vi "ElevatorSim_Execute.vi"(5 "LinearSystemID_Elevator_Model _Params":T7={"DCMOTOR_TYPES"=enum."NEO", "Num Motors"=1, "WinchRadias_Meters"=0.75, "mass_Kg"=26.0, "Gearing"=128.0} {"Gearing" format="%#_13g"; "mass_Kg" format="%#_13g"; "WinchRadias_Meters" format="%#_13g"}, 7 "ElevatorSim_Simulation _Params":T6={"MinHeight_Meters"=0.0, "MaxHeight_Meters"=0.0, "Measurment StdDev"=0.09, "SimulateGravity"=TRUE} {"Measurment StdDev" format="%#_13g"}, 8 "dT_Seconds":dbl=0.02 format="%#_13g", 10 "Battery Volts":dbl=12.0, 11 "Motor Dmd":dbl) -> (0 "Error":bool, 1 "AtLowLimit":bool, 2 "At HIgh LImit":bool, 3 "ElevatorHeight_Meters":dbl, 4 "Motor Current":dbl, 6 "out ElevatorSim":T1={"LinearSystemSim"={"m_Plant"={"m_A"=[], "m_B"=[], "m_C"=[], "m_D"=[], "States"=0, "Inputs"=0, "Outputs"=0}, "m_X"=[], "m_Y"=[], "m_U"=[], "MeasureStdDev"=[]}, "GearBox"={"nominalVoltage_Volts"=0.0, "StallTorque_NM"=0.0, "StallCurrent_Amps"=0.0, "FreeCurrent_Amps"=0.0, "FreeSpeed_RadPerSec"=0.0, "R_Ohms"=0.0, "KvINV_RadPerSecPerVolt"=0.0, "Kt_NMPerAmp"=0.0, "L_H"=0.0, "Jr_KgM2"=0.0}, "Gearing"=0.0, "DrumRadius_M"=0.0, "MinHeight_M"=0.0, "MaxHeight_M"=0.0, "CarriageMass_Kg"=0.0, "SimulateGravity"=TRUE} {"GearBox"."Jr_KgM2" format="%13.5p"; "GearBox"."L_H" format="%13.5p"; "GearBox"."Kt_NMPerAmp" format="%13.5p"; "GearBox"."KvINV_RadPerSecPerVolt" format="%13.5p"; "GearBox"."R_Ohms" format="%13.5p"; "GearBox"."FreeSpeed_RadPerSec" format="%13.5p"; "GearBox"."FreeCurrent_Amps" format="%13.5p"; "GearBox"."StallCurrent_Amps" format="%13.5p"; "GearBox"."StallTorque_NM" format="%13.5p"; "GearBox"."nominalVoltage_Volts" format="%13.5p"})   [LabVIEW 2019, in "Trajectory_Library.lvlib"]
doc: "Single call LabVIEW function to simulate an Elevatorr system. \n\nThe Elevator linear system definition is:\n - States\n - position (meters)\n - velocity (meters/sec)\n - Inputs:\n - motor voltage (volts)\n - Outputs:\n - position (meters)\n\n\nInputs:\n - LinearSystem Elevator Model Params -- cluster -- Contains physical configuration for Elevator system.\n - Elevator Sim Simulation Params -- cluster -- Contains siulation configuration.\n - Motor Dmd (CO) -- double -- motor demand value (+/- 1.0 )\n - Battery Voltage -- double -- Current simulated battery voltage (Volts)\n - dT Sec -- double -- Update period (Seconds, Default: 0.02)\n\nOutputs:\n - ElevatorHeight -- double -- Current elevator height (meters)\n - At High Limit -- boolean -- Elevator has reached high height limit\n - At Low Limit -- boolean -- Elevator has reached low height limit\n - Error -- boolean -- If TRUE an error occured.\n - Motor Current -- double -- Current motor current (Amps)\n - outElevatorSim -- cluster -- Current internal data cluster."
uses:
  Trajectory_Library.lvlib
  <vilib>/Analysis/Matrix/Datatypes/RealMatrix.ctl
  <vilib>/Analysis/Matrix/NI_Matrix.lvlib
  TypeDef/LINEAR_SYSTEM.ctl
  Enum/DCMOTOR_TYPES_ENUM.ctl
  TypeDef/LINEAR_SYSTEM_SIM.ctl
  TypeDef/DCMOTOR.CTL
  TypeDef/ELEVATOR_SIM.ctl
  TypeDef/LINEAR_SYSTEM_ID_ELEVATOR_MODEL.CTL
  TypeDef/ELEVATOR_SIM_SIMULATION_PARAMS.ctl
panel:
  out "Velocity_MetersPerSec":dbl
  # "<States, 1>"
  # "<Outputs, 1>"
  # "<Inputs, 1>"
  # "<Outputs, 1>"
  # "<States,States>"
  # "<States,Inputs>"
  # "<Outputs,States>"
  # "<Outputs,Inputs>"
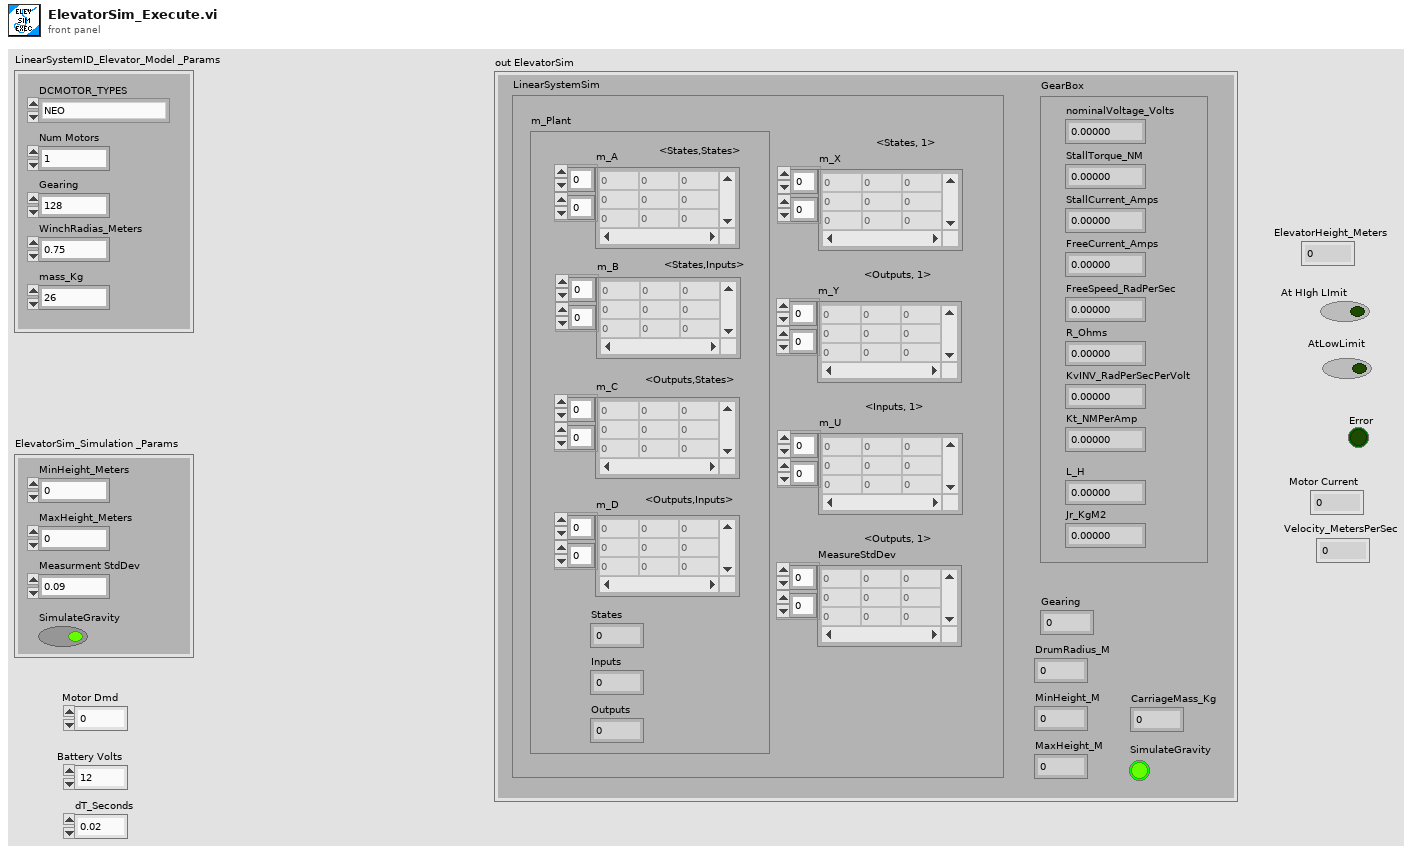
[diagram p1: front panel]
types:
  T1 = typedef "Trajectory_Library.lvlib/ELEVATOR_SIM.ctl" = cluster{"LinearSystemSim":T2, "GearBox":T5, "Gearing":dbl, "DrumRadius_M":dbl, "MinHeight_M":dbl, "MaxHeight_M":dbl, "CarriageMass_Kg":dbl, "SimulateGravity":bool}
  T2 = typedef "Trajectory_Library.lvlib/LINEAR_SYSTEM_SIM.ctl" = cluster{"m_Plant":T3, "m_X":T4, "m_Y":T4, "m_U":T4, "MeasureStdDev":T4}
  T3 = typedef "Trajectory_Library.lvlib/LINEAR_SYSTEM.ctl" = cluster{"m_A":T4, "m_B":T4, "m_C":T4, "m_D":T4, "States":i32, "Inputs":i32, "Outputs":i32}
  T4 = typedef "NI_Matrix.lvlib/RealMatrix.ctl" = dbl[][]
  T5 = typedef "Trajectory_Library.lvlib/DCMOTOR.CTL" = cluster{"nominalVoltage_Volts":dbl, "StallTorque_NM":dbl, "StallCurrent_Amps":dbl, "FreeCurrent_Amps":dbl, "FreeSpeed_RadPerSec":dbl, "R_Ohms":dbl, "KvINV_RadPerSecPerVolt":dbl, "Kt_NMPerAmp":dbl, "L_H":dbl, "Jr_KgM2":dbl}
  T6 = typedef "Trajectory_Library.lvlib/ELEVATOR_SIM_SIMULATION_PARAMS.ctl" = cluster{"MinHeight_Meters":dbl, "MaxHeight_Meters":dbl, "Measurment StdDev":dbl, "SimulateGravity":bool}
  T7 = typedef "Trajectory_Library.lvlib/LINEAR_SYSTEM_ID_ELEVATOR_MODEL.CTL" = cluster{"DCMOTOR_TYPES":T8, "Num Motors":i32, "WinchRadias_Meters":dbl, "mass_Kg":dbl, "Gearing":dbl}
  T8 = typedef "Trajectory_Library.lvlib/DCMOTOR_TYPES_ENUM.ctl" = enum16{"CIM", "AndyMark 9015", "Andy Mark RS 775 125", "Bag", "BaneBots RS 550", "BaneBots RS 775", "Falcon 500", "Mini CIM", "NEO", "NEO 550", "Romi BuiltIn", "Vex 775 Pro", "Snow Blower AM 2235A", "Bosch Seat AM 3493", "Falcon 500 FOC", "Kraken X60", "Kraken X60 FOC", "NEO Vortex"}
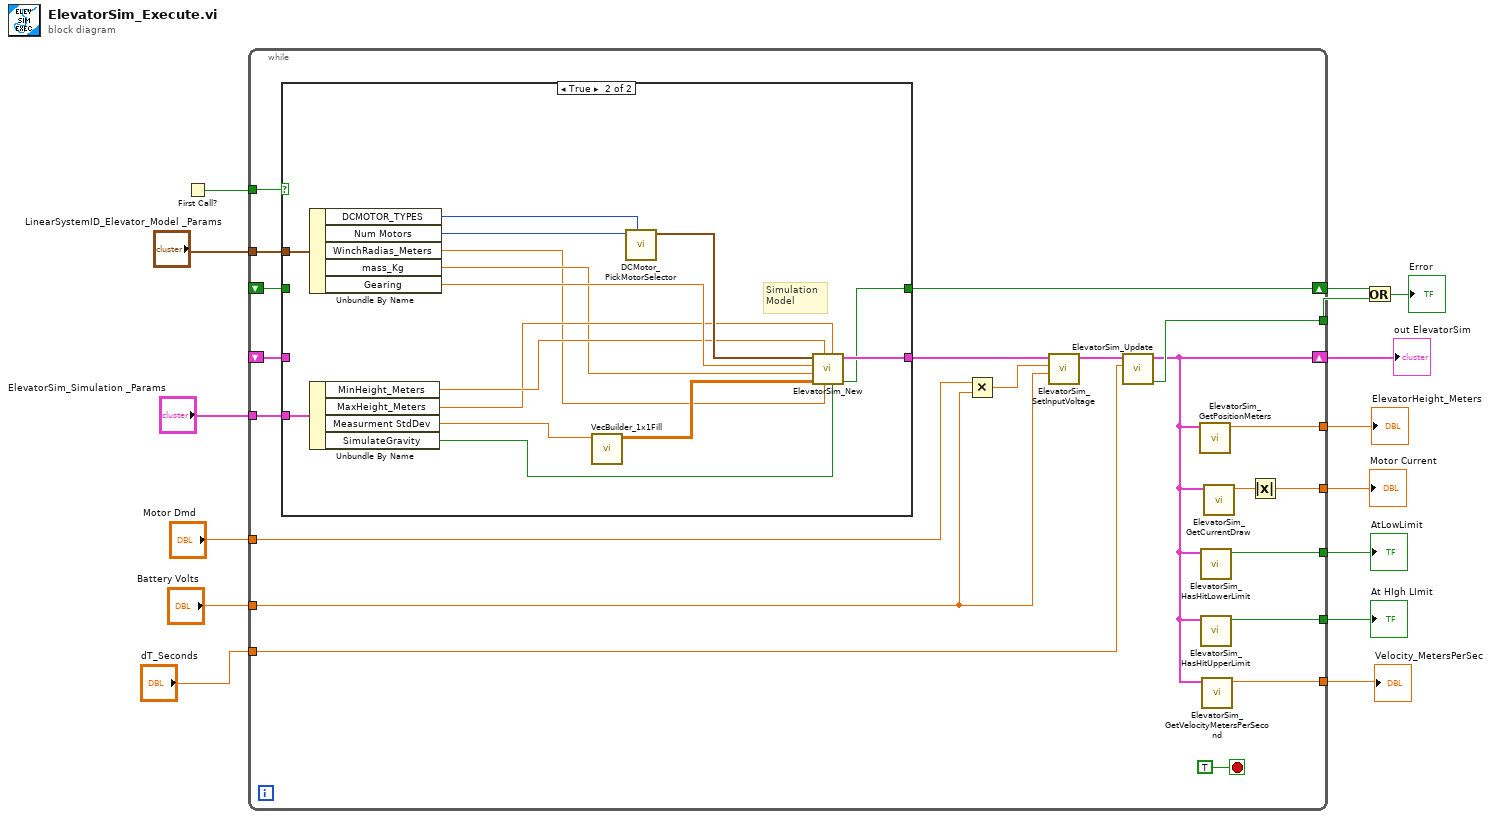
[diagram p0: block diagram]
diagram:
  n1 = First Call?() -> (First Call?: T/F=w14:bool)
  n2 = while {
    tunnel: "LinearSystemID_Elevator_Model _Params" -> [w36]
    tunnel: w14 -> [w35]
    shift-right: [w17] -> w2
    shift-left: _ -> [w34]
    shift-right: [w33] -> w7
    shift-left: _ -> [w32]
    tunnel: "Motor Dmd" -> [w27]
    tunnel: "Battery Volts" -> [w26]
    tunnel: [w25] -> w11
    tunnel: [w23] -> w10
    tunnel: [w22] -> w9
    tunnel: [w21] -> w8
    tunnel: [w20] -> w6
    tunnel: "dT_Seconds" -> [w19]
    tunnel: "ElevatorSim_Simulation _Params" -> [w18]
    tunnel: [w16] -> w1
    stop <- TRUE stop-if-true
    n3 = case shown="True" w35 {
      tunnel: [w38 w51] -> w28
      tunnel: w36 -> [_ w50]
      tunnel: w34 -> [w38 _]
      tunnel: [w37 w39] -> w33
      tunnel: w32 -> [w37 _]
      tunnel: w18 -> [_ w46]
      frame False {
      }
      frame True {
        # "Simulation \nModel"
        n4 = Unbundle By Name(w50) -> ("DCMOTOR_TYPES"=w47:T8, "Num Motors"=w48:i32, "WinchRadias_Meters"=w40:dbl, "mass_Kg"=w42:dbl, "Gearing"=w49:dbl)
        n5 = Unbundle By Name(w46) -> ("MinHeight_Meters"=w44:dbl, "MaxHeight_Meters"=w43:dbl, "Measurment StdDev"=w45:dbl, "SimulateGravity"=w41:bool)
        n6 = call "VecBuilder_1x1Fill.vi"("R0_C0"=w45) -> ("output matrix"=w53:T4)  [unwired: 10 in]
        n7 = call "DCMotor_PickMotorSelector.vi"("DCMOTOR_TYPES"=w47, "Num Motors"=w48) -> ("DCMOTOR"=w52:T5)  [unwired: 9 in]
        n8 = call "ElevatorSim_New.vi"("Simulate Gravity"=w41, "MaxHeight_Meters"=w43, "DrumRadius_Meters"=w40, "MinHeight_Meters"=w44, "MeasurementStdDev"=w53, "CarriageMass_Kg"=w42, "Gearing"=w49, "GearBox"=w52) -> ("Error"=w39:bool, "ElevatorSim"=w51:T1)  [unwired: 2 in]
      }
    }
    n9 = Multiply(x=w27, y=w26) -> (x*y=w31:dbl)
    n10 = call "ElevatorSim_SetInputVoltage.vi"("Battery_Volts"=w26, "Input_Voltage"=w31, "in ElevatorSim"=w28) -> ("out ElevatorSim"=w29:T1)  [unwired: 8 in]
    n11 = call "ElevatorSim_Update.vi"("dT_Seconds"=w19, "in ElevatorSim"=w29) -> ("Error"=w20:bool, "out ElevatorSim"=w17:T1)  [unwired: 8 in]
    n12 = call "ElevatorSim_GetPositionMeters.vi"("ElevatorSim"=w17) -> ("Position_Meters"=w23:dbl)  [unwired: 10 in]
    n13 = call "ElevatorSim_HasHitLowerLimit.vi"("ElevatorSim"=w17) -> ("AtLowLimit"=w21:bool)  [unwired: 10 in]
    n14 = call "ElevatorSim_HasHitUpperLimit.vi"("ElevatorSim"=w17) -> ("At HIgh LImit"=w22:bool)  [unwired: 10 in]
    n15 = call "ElevatorSim_GetVelocityMetersPerSecond.vi"("ElevatorSim"=w17) -> ("Velocity_MetersPerSec"=w16:dbl)  [unwired: 10 in]
    n16 = call "ElevatorSim_GetCurrentDraw.vi"("ElevatorSim"=w17) -> ("Current_Amps"=w30:dbl)  [unwired: 10 in]
    n17 = Absolute Value(x=w30) -> (abs(x)=w25:dbl)
  }
  "Motor Current" <- w11
  "ElevatorHeight_Meters" <- w10
  "AtLowLimit" <- w8
  "At HIgh LImit" <- w9
  "out ElevatorSim" <- w2
  "Velocity_MetersPerSec" <- w1
  n18 = Or(x=w7, y=w6) -> (x .or. y?=→"Error":bool)
